vi "Request_URL.vi"(8 "error in (no error)":errorcluster, 11 "LabVIEW Web Service Request":refnum<class "Web Request.lvclass">) -> (0 "error out":errorcluster, 2 "Request Origin":string, 3 "LabVIEW Web Service Request out":refnum<class "Web Request.lvclass">)   [LabVIEW 2015]
doc: "Obtains the request URL"
uses:
  <vilib>/wsapi/Web Request.lvclass
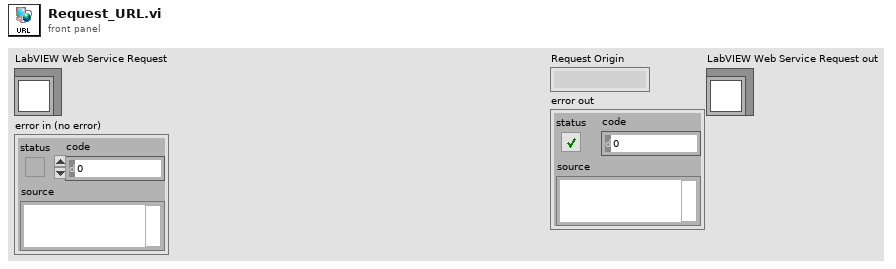
[diagram p1: front panel]
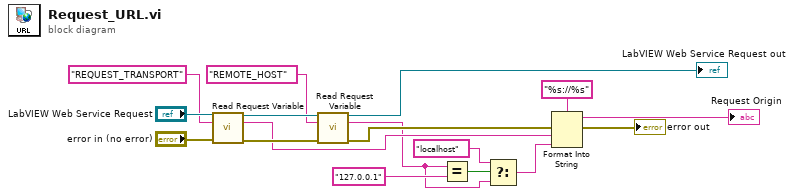
[diagram p0: block diagram]
diagram:
  n1 = call <vilib>:"Read Request Variable.vi"("LabVIEW Web Service Request"="LabVIEW Web Service Request", "variable name"="REQUEST_TRANSPORT", "error in (no error)"="error in (no error)") -> ("LabVIEW Web Service Request out"=w11:refnum<class "Web Request.lvclass">, "value"=w7:string, "error out"=w10:errorcluster)  [unwired: 10 in]
  n2 = call <vilib>:"Read Request Variable.vi"("LabVIEW Web Service Request"=w11, "variable name"="REMOTE_HOST", "error in (no error)"=w10) -> ("LabVIEW Web Service Request out"=→"LabVIEW Web Service Request out":refnum<class "Web Request.lvclass">, "value"=w2:string, "error out"=w6:errorcluster)  [unwired: 10 in]
  n3 = Equal?(x=w2, y="127.0.0.1") -> (x = y?=w5:bool)
  n4 = Select(t="localhost" ("y"), s=w5, f=w2) -> (s? t:f=w1:string)
  n5 = Format Into String(format string="%s://%s", error in=w6, w7, w1) -> (resulting string=→"Request Origin":string, error out=→"error out":errorcluster)  [unwired: 1 in]
